vi "Get Next Value from Attribute List.vi"(7 "element name (for errors)":string, 8 "error in":errorcluster, 9 "offset":i32, 11 "attribute list":string) -> (0 "error out":errorcluster, 1 "offset past value and whitespace":i32, 2 "value":string)   [LabVIEW 2011]
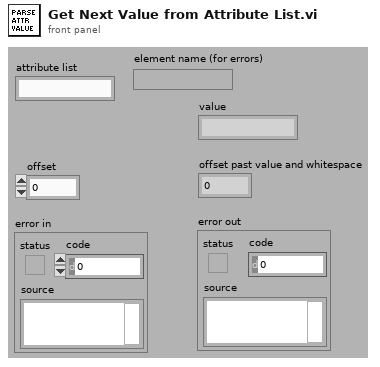
[diagram p1: front panel]
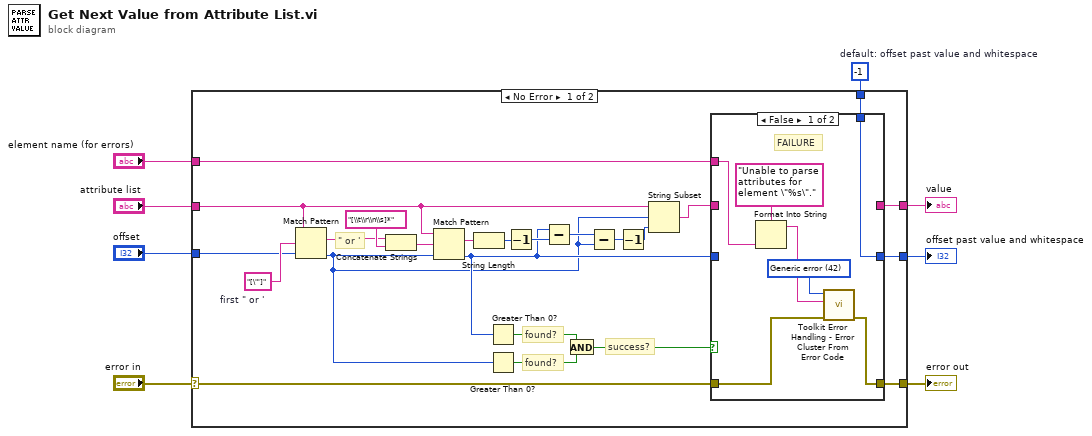
[diagram p0: block diagram]
diagram:
  w2 = -1  # default: offset past value and whitespace
  n1 = case shown="No Error" "error in" {
    selector: "error in" -> [w20 w44]
    tunnel: [w11 _] -> w3
    tunnel: [w17 w43] -> w4
    tunnel: "offset" -> [w29 _]
    tunnel: "attribute list" -> [w28 _]
    tunnel: [w19 w44] -> w8
    tunnel: w2 -> [w18 w43]
    tunnel: "element name (for errors)" -> [w10 _]
    frame No Error {
      w32 = "[\"']"  # first " or '
      # "found?"
      # "found?"
      # "success?"
      # "\" or '"
      n2 = Match Pattern(string=w28, regular expression=w32, offset (0)=w29) -> (match substring=w26:string, offset past match=w9:i32)  [unwired: 2 out]
      n3 = Concatenate Strings(w26, "[\\t\\r\\n\\s]*" ("regular expression")) -> (w25:string)
      n4 = Match Pattern(string=w28, regular expression=w25, offset (0)=w9) -> (match substring=w24:string, offset past match=w13:i32)  [unwired: 2 out]
      n5 = String Length(string=w24) -> (length=w23:i32)
      n6 = Greater Than 0?(x=w13) -> (x > 0?=w15:bool)
      n7 = Greater Than 0?(x=w9) -> (x > 0?=w14:bool)
      n8 = Decrement(x=w23) -> (x-1=w21:i32)
      n9 = Subtract(x=w13, y=w21) -> (x-y=w22:i32)
      n10 = And(x=w15, y=w14) -> (x .and. y?=w12:bool)
      n11 = Subtract(x=w22, y=w9) -> (x-y=w31:i32)
      n12 = Decrement(x=w31) -> (x-1=w30:i32)
      n13 = String Subset(string=w28, offset (0)=w9, length (rest)=w30) -> (substring=w16:string)
      n14 = case shown="False" w12 {
        tunnel: [_ w42] -> w11
        tunnel: w16 -> [_ w42]
        tunnel: [w39 w41] -> w17
        tunnel: w13 -> [_ w41]
        tunnel: w20 -> [w38 w40]
        tunnel: [w37 w40] -> w19
        tunnel: w18 -> [w39 _]
        tunnel: w10 -> [w35 _]
        frame False {
          w36 = 42 items=["No error", "Argument error", "Memory is full", "Out of zone", "End of file", "File already open", "Generic file I/O error", "File not found", "File permission error", "Disk is full", "Duplicate path", "Too many files open", "System feature not enabled", "Resource file not found", "Cannot add resource", "Resource not found", "Image not found", "Image memory error", "Pen does not exist", "Config type invalid", "Config token not found", "Config parse error", "Config memory error", "Bad external code format", "Bad external code offset", "External code not present", "Null window", "Destroy window error", "Null menu", "Print aborted", "Bad print record", "Print driver error", "Windows error during printing", "Memory error during printing", "Print dialog error", "Generic print error", "Invalid device refnum", "Device not found", "Device parameter error", "Device unit error", "Cannot open device", "Device call aborted", "Generic error", "Cancelled by user", "Object ID too low", "Object ID too high", "Object not in heap", "Unknown heap", "Unknown object (invalid DefProc)", "Unknown object (DefProc not in table)", "Message out of range", "Invalid (null) method", "Unknown message", "Manager call not supported", "Bad address", "Network operation in progress", "Network operation timed out", "Connection is busy", "Network attribute not supported", "Network error", "Address in use", "System out of memory", "Connection aborted", "Connection refused", "Not connected", "Already connected", "Connection closed", "Initialization error (interapplication manager)", "Bad occurrence", "Wait on unbound occurrence handler", "Occurrence queue overflow", "Datalog type conflict", "Unused", "Unrecognized type (interapplication manager)", "Memory corrupt", "Failed to make temporary DLL", "Old CIN version", "Drag socket not found", "Failed to load drop-object", "Failed to register OLE object", "Failed to release OLE object", "Format specifier type mismatch", "Unknown format specifier", "Too few format specifiers", "Too many format specifiers", "Scan failed", "Newer CIN version", "Error converting to variant", "Runtime menu error", "Password tampered", "Variant attribute not found", "Incompatible variant data type", "Event data is not available", "Event Store is not present", "Occurrence is not found", "Event Queue is not created", "Event info is not available", "Refnum passed is NULL", "Error retrieving Class GUID", "Error retrieving CoClass GUID", "Error retrieving TypeLib GUID.", "Bad built application magic bytes.", "Specific driver is different from the specific driver associated with the Logical Name.", "There is no session opened to the class driver.", "Max Error", "MAX - Error with config objects", "MAX - Error loading configuration", "MAX - Group not supported"]
          # "FAILURE"
          n15 = Format Into String(format string="Unable to parse attributes for element \"%s\".", w35) -> (resulting string=w33:string)  [unwired: 2 in, 1 out]
          n16 = call "Toolkit Error Handling - Error Cluster From Error Code.vi"("error in"=w38, "error message (\"\")"=w33, "error code (0)"=w36) -> ("error out"=w37:errorcluster)  [unwired: 6 in]
        }
        frame True {
          # "SUCCESS"
        }
      }
    }
    frame Error {
    }
  }
  "error out" <- w8
  "offset past value and whitespace" <- w4
  "value" <- w3
